vi "Read Position.vi"(8 "error in (no error)":errorcluster, 10 "No. of attempts":i32=3, 11 "XYZ Stage Control in":refnum<class "XYZ Stage Control.lvclass">) -> (0 "error out":errorcluster, 1 "No Feedback":bool, 2 "Stage XYZ Position":cluster{"X":sgl, "Y":sgl, "Z":sgl}, 3 "XYZ Stage Control out":refnum<class "XYZ Stage Control.lvclass">)   [LabVIEW 2020, in "TranslationStageClassStructure.lvlib" / "XYZ Stage Control.lvclass"]
uses:
  XYZ Stage Control.lvclass
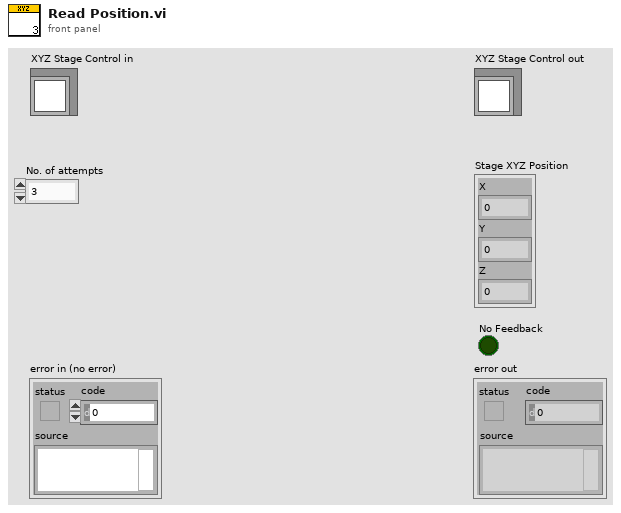
[diagram p1: front panel]
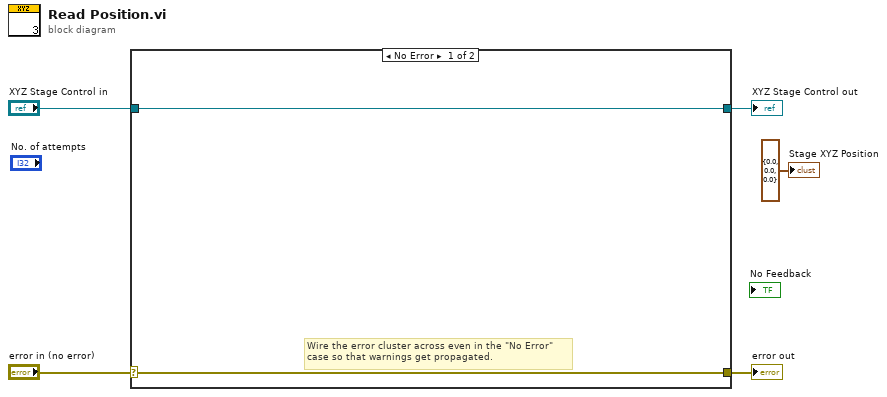
[diagram p0: block diagram]
diagram:
  n1 = case shown="No Error" "error in (no error)" {
    selector: "error in (no error)" -> [w6 w9]
    tunnel: [w6 w9] -> w4
    tunnel: [w7 w8] -> w2
    tunnel: "XYZ Stage Control in" -> [w7 w8]
    frame No Error {
      # "Wire the error cluster across even in the \"No Error\"\ncase so that warnings get propagated."
    }
    frame Error {
    }
  }
  "error out" <- w4
  "XYZ Stage Control out" <- w2
  "Stage XYZ Position" <- cluster{"X":sgl, "Y":sgl, "Z":sgl} {"X"=0.0, "Y"=0.0, "Z"=0.0} ("Stage XYZ Position")
